vi "VCM_read_values.vi"(4 "mode":u16(ring), 5 "delay time":dbl, 6 "address":string) -> (1 "Frequenz IST":dbl, 2 "Amplitude IST":dbl)   [LabVIEW 2019]
panel:
  out "Y 3":string="1.298E-05\r\n"
  out "Y 4":string="1.298E-05\r\n"
  in  "read GPIB (false=on) 4":bool
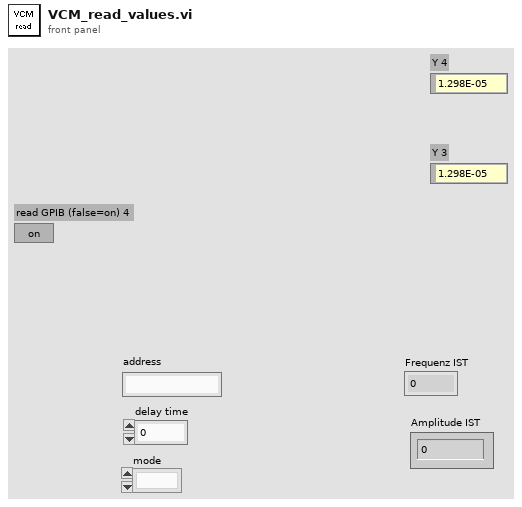
[diagram p1: front panel]
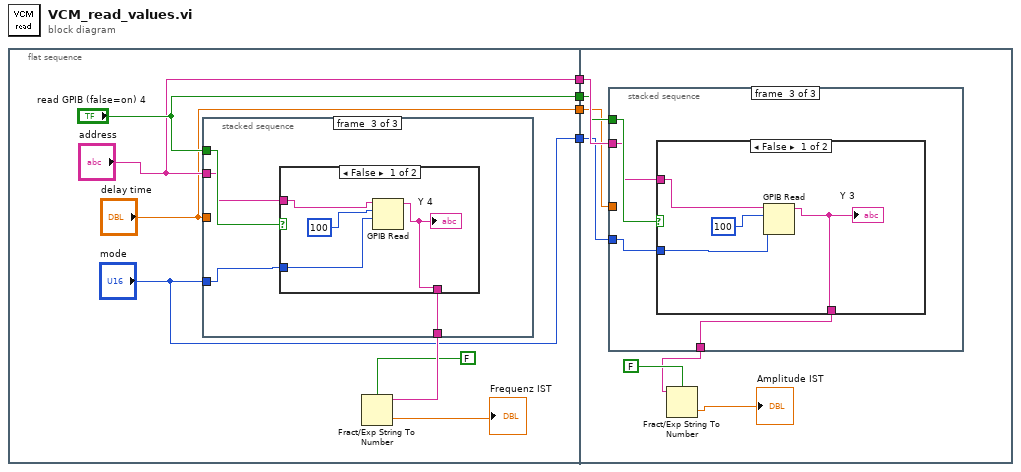
[diagram p0: block diagram]
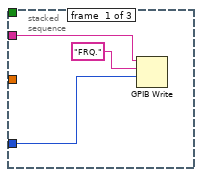
[diagram p2: hidden frame]
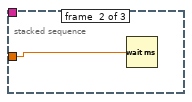
[diagram p3: hidden frame]
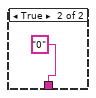
[diagram p4: hidden frame]
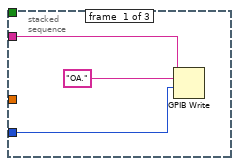
[diagram p5: hidden frame]
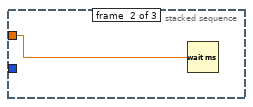
[diagram p6: hidden frame]
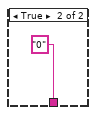
[diagram p7: hidden frame]
diagram:
  n1 = flat-sequence {
    tunnel: ["read GPIB (false=on) 4"] -> w4
    tunnel: ["address"] -> w3
    tunnel: ["delay time"] -> w2
    tunnel: ["mode"] -> w1
    tunnel: w4 -> [w30]
    tunnel: w3 -> [w31]
    tunnel: w2 -> [w29]
    tunnel: w1 -> [w28]
    frame #0 {
      n2 = stacked-sequence {
        tunnel: "address" -> [w14 _ w18]
        tunnel: "delay time" -> [_ w15 _]
        tunnel: "mode" -> [w13 _ w17]
        tunnel: "read GPIB (false=on) 4" -> [_ _ w19]
        tunnel: [_ _ w16] -> w11
        frame #0 {
          n3 = GPIB Write(0:w14, 1:"FRQ.", 2:w13) -> ()  [unwired: 2 in, 2 out]
        }
        frame #1 {
          n4 = Wait (ms)(milliseconds to wait=w15) -> ()  [unwired: 1 out]
        }
        frame #2 {
          n5 = case shown="False" w19 {
            tunnel: w18 -> [w23 _]
            tunnel: w17 -> [w22 _]
            tunnel: [w20 "0"] -> w16
            frame False {
              n6 = GPIB Read(0:w23, 1:100, 2:w22) -> (5:w20:string)  [unwired: 2 in, 2 out]
              "Y 4" <- w20
            }
            frame True {
            }
          }
        }
      }
      n7 = Fract/Exp String To Number(use system decimal point (T)=FALSE, string=w11) -> (number=→"Frequenz IST":dbl)  [unwired: 2 in, 1 out]
    }
    frame #1 {
      n8 = stacked-sequence {
        tunnel: w31 -> [w34 _ w38]
        tunnel: w30 -> [_ _ w39]
        tunnel: w29 -> [_ w35 _]
        tunnel: w28 -> [w33 _ w37]
        tunnel: [_ _ w36] -> w26
        frame #0 {
          n9 = GPIB Write(0:w34, 1:"OA.", 2:w33) -> ()  [unwired: 2 in, 2 out]
        }
        frame #1 {
          n10 = Wait (ms)(milliseconds to wait=w35) -> ()  [unwired: 1 out]
        }
        frame #2 {
          n11 = case shown="False" w39 {
            tunnel: w38 -> [w43 _]
            tunnel: w37 -> [w42 _]
            tunnel: [w40 "0"] -> w36
            frame False {
              n12 = GPIB Read(0:w43, 1:100, 2:w42) -> (5:w40:string)  [unwired: 2 in, 2 out]
              "Y 3" <- w40
            }
            frame True {
            }
          }
        }
      }
      n13 = Fract/Exp String To Number(use system decimal point (T)=FALSE, string=w26) -> (number=→"Amplitude IST":dbl)  [unwired: 2 in, 1 out]
    }
  }
